vi "AlliGator Check .bin File Type.vi"(8 "error in (no error)":errorcluster, 11 "File Path":path) -> (0 "error out":errorcluster, 1 "Folder Selection Mode":T1, 2 "bin FLI Dataset Type":T2, 3 "File Path dup":path)   [LabVIEW 2021, in "AlliGator Files.lvlib"]
doc: "Determines what type of binned dataset image this is (PicoQuant or EPFL Piccolo)."
uses:
  AlliGator Files.lvlib
  AlliGator FLI Dataset Type.ctl
  AlliGator Select Folder Mode.ctl
  PicoQuant/PicoQuant.lvlib
panel:
  # "see the AlliGator License on the block diagram (Ctrl+E or Window:Show Block Diagram)"
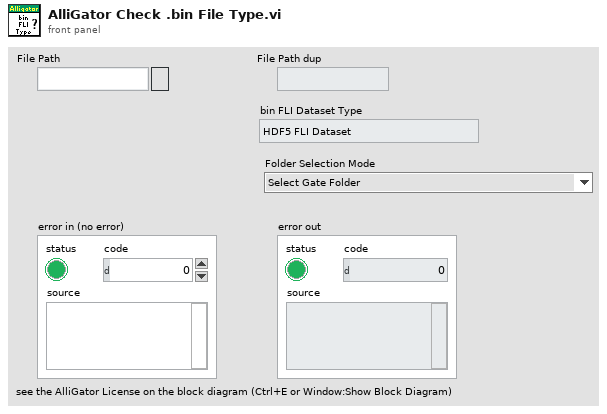
[diagram p1: front panel]
types:
  T1 = typedef "AlliGator Files.lvlib/AlliGator Select Folder Mode.ctl" = enum16{"Select Gate Folder", "Select Folder of Gate Folders", "Select Folder of SwissSPAD 2 Datasets", "Select Folder of .sdt FLI Datasets (Becker & Hickl)", "Select Folder of .ptu FLI Datasets (PicoQuant)", "Select Folder of .bin FLI Datasets (PicoQuant Binned)", "Select Folder of .bin FLI Datasets (Piccolo Binned)", "Select Folder of HDF5 FLI Datasets"}
  T2 = typedef "AlliGator Files.lvlib/AlliGator FLI Dataset Type.ctl" = enum16{"HDF5 FLI Dataset", "Gate Image Folder", ".sdt FLI Dataset (Becker & Hickl)", ".ptu FLI Dataset (PicoQuant)", "SS1 FLI Dataset", "SS2 FLI Dataset", "I/m/phi Dataset", ".bin FLI Dataset (PicoQuant Binned)", ".bin FLI Dataset (Piccolo Binned)"}
  T3 = typedef "PicoQuant.lvlib/BIN File Information.ctl" = cluster{"# Pixels X":i32, "# Pixels Y":i32, "Spatial Resolution":dbl[unit], "# TCSPC Bins":i32, "Temporal Resolution":dbl[unit]}
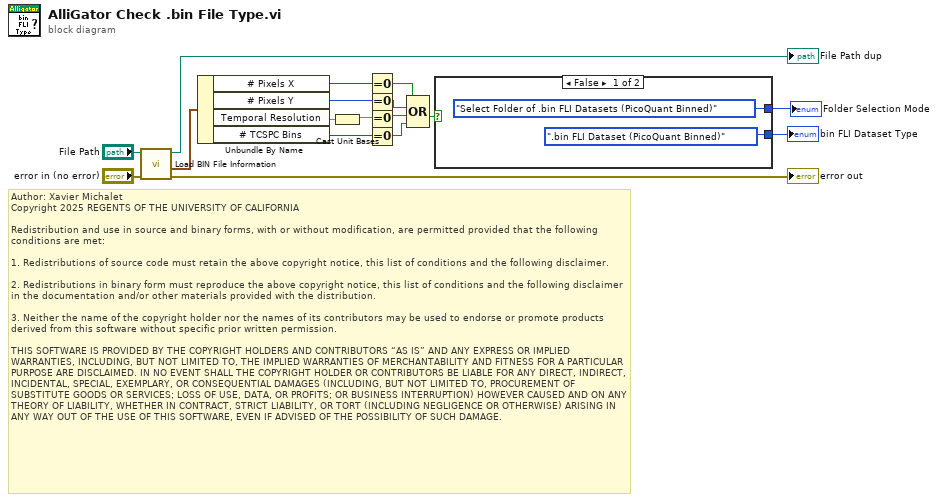
[diagram p0: block diagram]
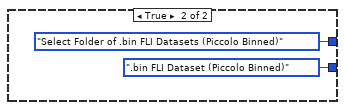
[diagram p2: hidden frame]
diagram:
  # "Author: Xavier Michalet\nCopyright 2025 REGENTS OF THE UNIVERSITY OF CALIFORNIA\n\nRedistribution and use in source and binary forms, with or without modification, are permitted provided that the following conditions are met:\n\n1. Redistributions of source code must retain the above copyright notice, this list of conditions and the following disclaimer.\n\n2. Redistributions in binary form must reproduce the above copyright notice, this list of conditions and the following disclaimer in the documentation and/or other materials provided with the distribution.\n\n3. Neither the name of the copyright holder nor the names of its contributors may be used to endorse or promote products derived from this software without specific prior written permission.\n\nTHIS SOFTWARE IS PROVIDED BY THE COPYRIGHT HOLDERS AND CONTRIBUTORS “AS IS” AND ANY EXPRESS OR IMPLIED WARRANTIES, INCLUDING, BUT NOT LIMITED TO, THE IMPLIED WARRANTIES OF MERCHANTABILITY AND FITNESS FOR A PARTICULAR PURPOSE ARE DISCLAIMED. IN NO EVENT SHALL THE COPYRIGHT HOLDER OR CONTRIBUTORS BE LIABLE FOR ANY DIRECT, INDIRECT, INCIDENTAL, SPECIAL, EXEMPLARY, OR CONSEQUENTIAL DAMAGES (INCLUDING, BUT NOT LIMITED TO, PROCUREMENT OF SUBSTITUTE GOODS OR SERVICES; LOSS OF USE, DATA, OR PROFITS; OR BUSINESS INTERRUPTION) HOWEVER CAUSED AND ON ANY THEORY OF LIABILITY, WHETHER IN CONTRACT, STRICT LIABILITY, OR TORT (INCLUDING NEGLIGENCE OR OTHERWISE) ARISING IN ANY WAY OUT OF THE USE OF THIS SOFTWARE, EVEN IF ADVISED OF THE POSSIBILITY OF SUCH DAMAGE."
  n1 = call "Load BIN File Information.vi"("error in (no error)"="error in (no error)", "File Path"="File Path") -> ("error out"=→"error out":errorcluster, "BIN dataset Information"=w7:T3, "File Path out"=→"File Path dup":path)  [unwired: 4 in, 3 out]
  n2 = Unbundle By Name(w7) -> ("# Pixels X"=w9:i32, "# Pixels Y"=w10:i32, "Temporal Resolution"=w8:dbl[unit], "# TCSPC Bins"=w12:i32)
  n3 = Cast Unit Bases(0:w8) -> (2:w11:dbl)  [unwired: 1 in]
  n4 = Equal To 0?(x=w9) -> (x = 0?=w13:bool)
  n5 = Equal To 0?(x=w10) -> (x = 0?=w14:bool)
  n6 = Equal To 0?(x=w11) -> (x = 0?=w15:bool)
  n7 = Equal To 0?(x=w12) -> (x = 0?=w16:bool)
  n8 = Compound Arithmetic op=OR(w13, w14, w15, w16) -> (w17:bool)
  n9 = case shown="False" w17 {
    tunnel: [AlliGator_FLI_Dataset_Type.".bin FLI Dataset (PicoQuant Binned)" ("FLI Dataset Type") AlliGator_FLI_Dataset_Type.".bin FLI Dataset (Piccolo Binned)" ("FLI Dataset Type")] -> w2
    tunnel: [AlliGator_Select_Folder_Mode."Select Folder of .bin FLI Datasets (PicoQuant Binned)" ("Folder Selection Mode") AlliGator_Select_Folder_Mode."Select Folder of .bin FLI Datasets (Piccolo Binned)" ("Folder Selection Mode")] -> w1
    frame False {
    }
    frame True {
    }
  }
  "bin FLI Dataset Type" <- w2
  "Folder Selection Mode" <- w1
